vi "Check AttendanceTable If Correct.vi"(6 "CurWeek(0)":i32, 8 "error in (no error)":errorcluster, 9 "SheetName(\"\")":string="测试", 10 "Path":path, 11 "ExcelReader in":refnum<class "ExcelReader.lvclass">) -> (0 "error out":errorcluster, 2 "Fit(False)":bool, 3 "ExcelReader out":refnum<class "ExcelReader.lvclass">)   [LabVIEW 2015, in "Admin_Actor.lvlib" / "ExcelReader.lvclass"]
uses:
  ExcelReader.lvclass
  Setting/g_setting.vi
  CalAttendance/CalAttendance.lvclass
  Admin_Actor.lvlib
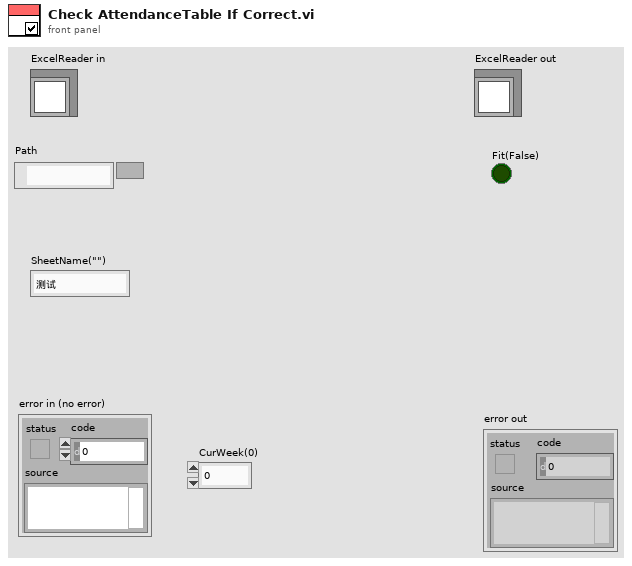
[diagram p1: front panel]
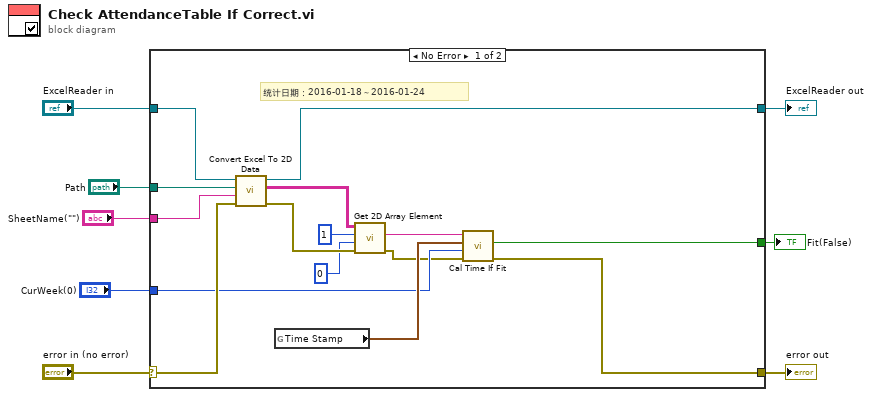
[diagram p0: block diagram]
diagram:
  n1 = case shown="No Error" "error in (no error)" {
    selector: "error in (no error)" -> [w20 w25]
    tunnel: [w10 w25] -> w7
    tunnel: [w15 w24] -> w5
    tunnel: "ExcelReader in" -> [w23 w24]
    tunnel: "Path" -> [w22 _]
    tunnel: "SheetName(\"\")" -> [w21 _]
    tunnel: "CurWeek(0)" -> [w12 _]
    tunnel: [w9 _] -> w1
    frame No Error {
      # "统计日期：2016-01-18～2016-01-24"
      n2 = call "Convert Excel To 2D Data.vi"("error in (no error)"=w20, "SheetName(\"\")"=w21, "Path"=w22, "ExcelReader in"=w23) -> ("error out"=w18:errorcluster, "data"=w19:string[][], "ExcelReader out"=w15:refnum<class "ExcelReader.lvclass">)  [unwired: 5 in]
      n3 = global read "g_setting.vi" "Time Stamp"() -> (w13:timestamp)
      n4 = call "Get 2D Array Element.vi"("error in (no error)"=w18, "Col"=0, "Row"=1, "Array"=w19) -> ("error out"=w11:errorcluster, "String"=w14:string)  [unwired: 5 in, 1 out]
      n5 = call "Cal Time If Fit.vi"("error in (no error)"=w11, "CurWeek(0)"=w12, "StandardStartTime"=w13, "Source Time(\"\")"=w14) -> ("error out"=w10:errorcluster, "Fit(False)"=w9:bool)  [unwired: 6 in]
    }
    frame Error {
    }
  }
  "error out" <- w7
  "ExcelReader out" <- w5
  "Fit(False)" <- w1
